vi "TESTING DUMMY PLC.vi"(8 "error in (no error)":errorcluster) -> (0 "error out":errorcluster, 3 "PLC Simu OUT":T1[](array[typedef]))   [LabVIEW 2017]
uses:
  Control/Main_Data.ctl
panel:
  in  "Array":T1[](array[typedef])
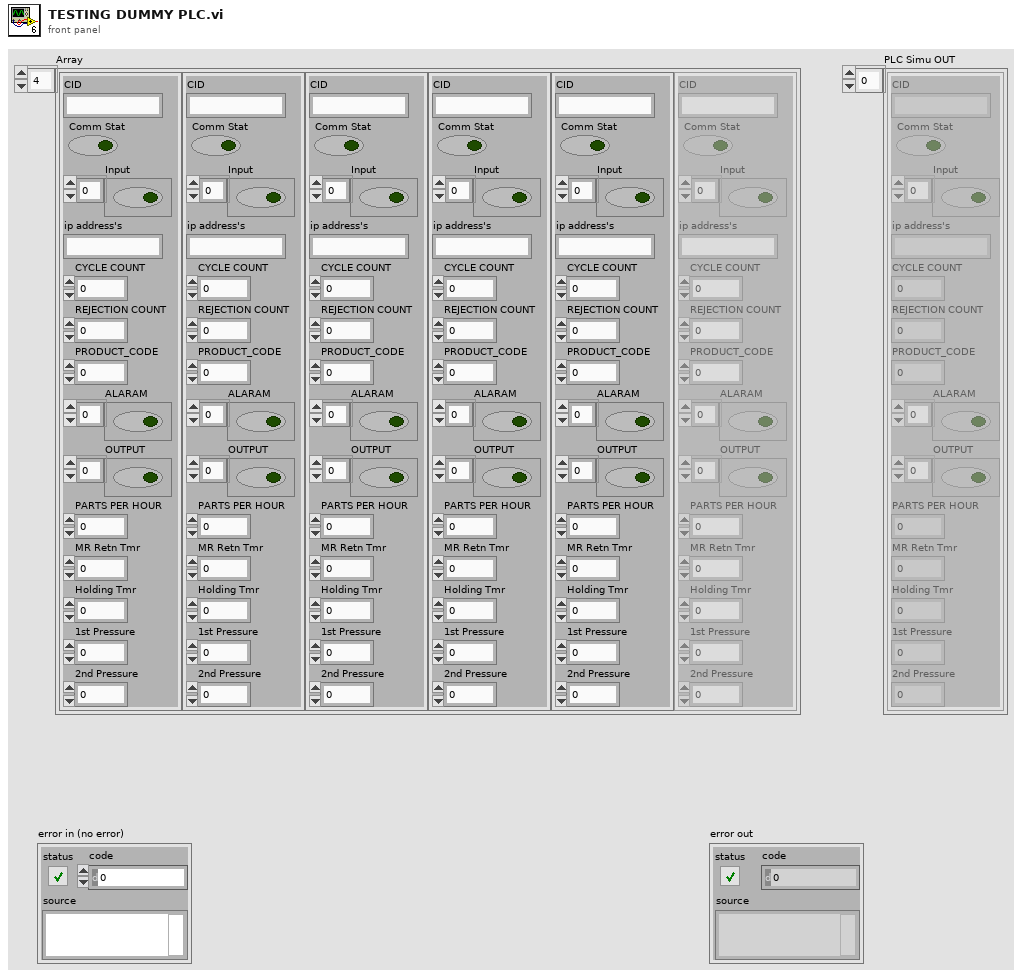
[diagram p1: front panel]
types:
  T1 = typedef "Main_Data.ctl" = cluster{"CID":string, "Comm Stat":bool, "Input":bool[], "ip address's":string, "CYCLE COUNT":u32, "REJECTION COUNT":u32, "PRODUCT_CODE":i16, "ALARAM":bool[], "OUTPUT":bool[], "PARTS PER HOUR":i16, "MR Retn Tmr":dbl, "Holding Tmr":dbl, "1st Pressure":dbl, "2nd Pressure":dbl}
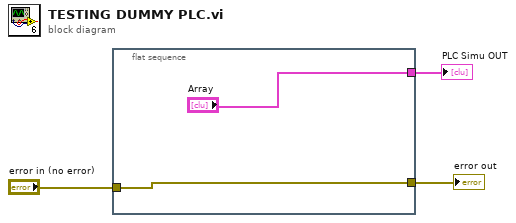
[diagram p0: block diagram]
diagram:
  n1 = flat-sequence {
    tunnel: [w5] -> w3
    tunnel: "error in (no error)" -> [w5]
    tunnel: ["Array"] -> w1
    frame #0 {
    }
  }
  "error out" <- w3
  "PLC Simu OUT" <- w1
